vi "Control Panel.vi"(8 "error in (no error)":errorcluster, 11 "Spectrometer Digikröm.lvclass in":refnum<class "Spectrometer Digikröm.lvclass">) -> (0 "error out":errorcluster, 3 "Spectrometer Digikröm.lvclass out":refnum<class "Spectrometer Digikröm.lvclass">)   [LabVIEW 2009, in "Spectrometer Digikröm.lvclass"]
uses:
  Spectrometer Digikröm.lvclass
  <vilib>/Utility/error.llb/DialogType.ctl
  Digikrom DK24x/Digikrom DK24x.lvlib
panel:
  in  "exit":bool
  in  "Control":T1={"Goto Wavelength"=0.0, "Slit 1 width"=1.0000000000000004e-05, "Slit 2 width"=1.0000000000000004e-05, "Filter"=3, "Grating"=1} {"Grating" items=["Grating A"=1, "Grating B"=2, "Grating C"=3]; "Filter" items=["No filter", "Filter 1", "Filter 2", "Filter 3", "Filter 4", "Filter 5", ""]; "Slit 2 width" min=1.0000000000000004e-05 max=0.005000000000000002 step=1.0000000000000004e-05; "Slit 1 width" min=1.0000000000000004e-05 max=0.005000000000000002 step=1.0000000000000004e-05; "Goto Wavelength" min=0.0 max=6e-06 step=1.0000000000000008e-13 format="%.2f"}
  out "Status":T2={"Ready"=FALSE, "Wavelength"=5.000000000000003e-07, "Entrance slit"=9.999999999999999e-06, "Exit slit"=9.999999999999999e-06, " Grating (nm)"=500.0, " Filter"=0.0} {"Exit slit" format="%.2f"; "Entrance slit" format="%.2f"; "Wavelength" min=0.0 format="%.2f"}
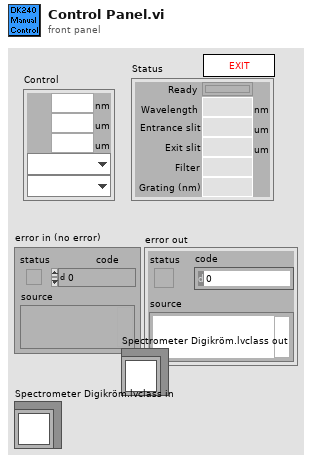
[diagram p1: front panel]
types:
  T1 = cluster{"Goto Wavelength":dbl[unit], "Slit 1 width":dbl[unit], "Slit 2 width":dbl[unit], "Filter":u32, "Grating":u16}
  T2 = cluster{"Ready":bool, "Wavelength":dbl[unit], "Entrance slit":dbl[unit], "Exit slit":dbl[unit], " Grating (nm)":dbl, " Filter":dbl}
  T3 = typedef "DialogType.ctl" = u16
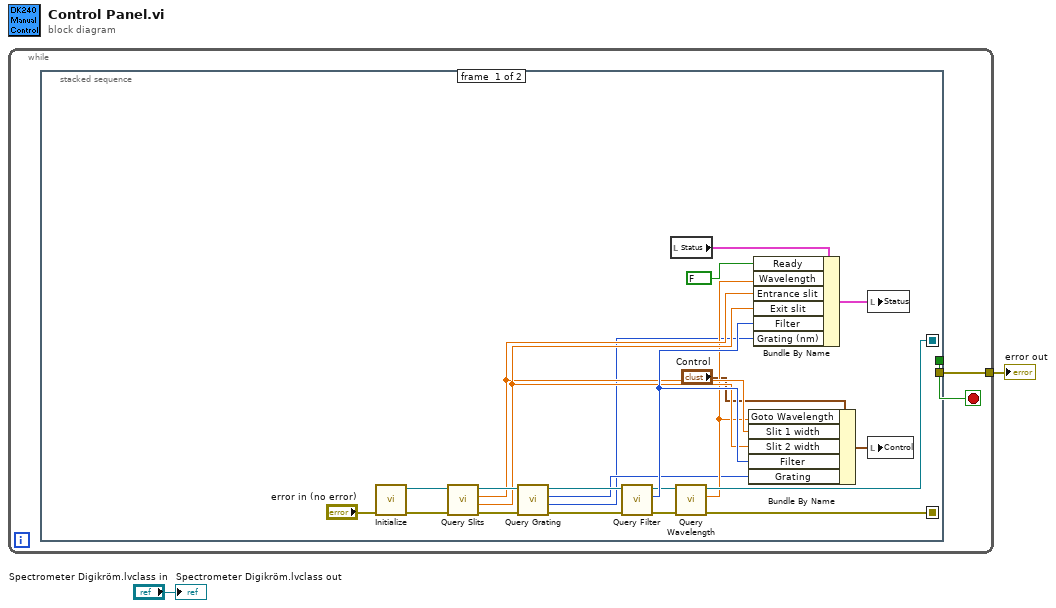
[diagram p0: block diagram]
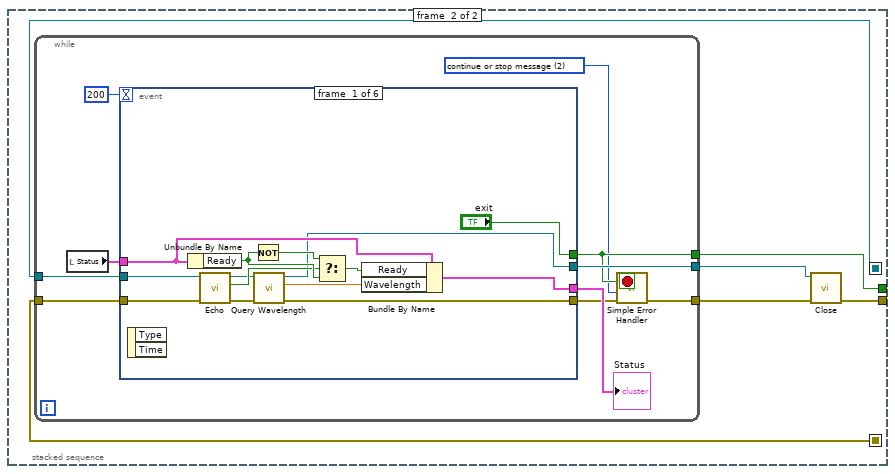
[diagram p2: hidden frame]
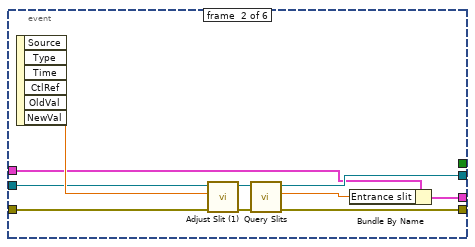
[diagram p3: hidden frame]
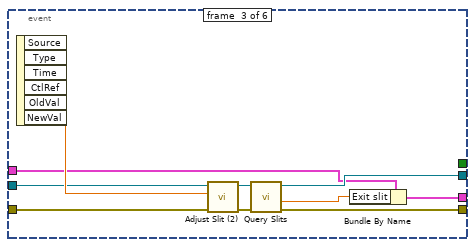
[diagram p4: hidden frame]
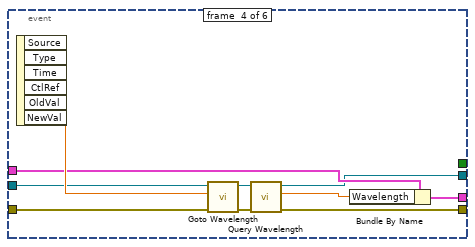
[diagram p5: hidden frame]
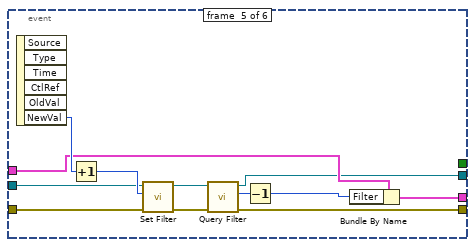
[diagram p6: hidden frame]
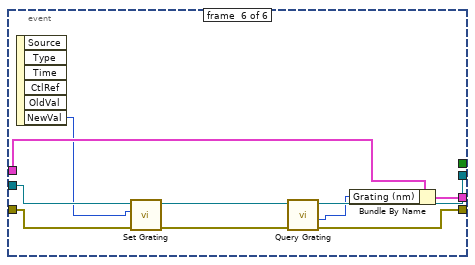
[diagram p7: hidden frame]
diagram:
  n1 = while {
    tunnel: [w3] -> w2
    stop <- w4 stop-if-true
    n2 = stacked-sequence {
      seq-local: [w19 _] -> [_ w31]
      seq-local: [w18 _] -> [_ w32]
      tunnel: [_ w30] -> w4
      tunnel: [_ w27] -> w3
      frame #0 {
        n3 = call "Initialize.vi"("error in (no error)"="error in (no error)") -> ("error out"=w23:errorcluster, "VISA resource name out"=w22:refnum<visa-resource-name>)  [unwired: 2 in, 7 out]
        n4 = call "Query Slits.vi"("error in (no error)"=w23, "VISA resource name"=w22) -> ("error out"=w20:errorcluster, "CURRENT S2 WIDTH"=w15:dbl[unit], "CURRENT S1 WIDTH"=w14:dbl[unit], "VISA resource name out"=w21:refnum<visa-resource-name>)  [unwired: 6 out]
        n5 = call "Query Grating.vi"("error in (no error)"=w20, "VISA resource name"=w21) -> ("error out"=w9:errorcluster, "BLAZE (nm)"=w7:u16, "GRATING #"=w8:u8, "VISA resource name out"=w10:refnum<visa-resource-name>)  [unwired: 6 out]
        n6 = call "Query Filter.vi"("error in (no error)"=w9, "VISA resource name"=w10) -> ("error out"=w11:errorcluster, "CURRENT FILTER"=w16:u8, "VISA resource name out"=w12:refnum<visa-resource-name>)  [unwired: 7 out]
        n7 = local read "Status"() -> (w25:T2)
        n8 = call "Query Wavelength.vi"("error in (no error)"=w11, "VISA resource name"=w12) -> ("error out"=w18:errorcluster, "CURRENT WAVELENGTH"=w13:dbl[unit], "VISA resource name out"=w19:refnum<visa-resource-name>)  [unwired: 7 out]
        n9 = Bundle By Name(cluster="Control", "Goto Wavelength"=w13, "Slit 1 width"=w14, "Slit 2 width"=w15, "Filter"=w16, "Grating"=w8) -> (w24:T1)
        n10 = Bundle By Name(cluster=w25, "Ready"=FALSE, "Wavelength"=w13, "Entrance slit"=w14, "Exit slit"=w15, "Filter"=w16, "Grating (nm)"=w7) -> (w26:T2)
        n11 = local write "Status"(w26) -> ()
        n12 = local write "Control"(w24) -> ()
      }
      frame #1 {
        n13 = while {
          tunnel: [w35] -> w30
          tunnel: w32 -> [w40]
          tunnel: [w34] -> w29
          tunnel: w31 -> [w39]
          tunnel: [w38] -> w28
          stop <- w35 stop-if-true
          w33 = T3 2 items=["no dialog", "OK message", "continue or stop message", "OK message + warnings", "continue/stop + warnings"] ("type of dialog (OK msg:1)")
          n14 = local read "Status"() -> (w36:T2)
          n15 = event shown="[5] \"Control.Grating\": Value Change" {
            selector: _ -> [_ _ _ _ _ _]
            dyn-events: _ -> [_ _ _ _ _ _]
            timeout: 200 -> [_ _ _ _ _ _]
            tunnel: ["exit" _ _ _ _ _] -> w35
            tunnel: [w56 w66 w76 w85 w97 w108] -> w42
            tunnel: w39 -> [w51 w60 w71 w82 w89 w107]
            tunnel: w40 -> [w52 w61 w72 w83 w93 w106]
            tunnel: [w46 w63 w74 w78 w87 w99] -> w37
            tunnel: [w47 w64 w75 w77 w88 w101] -> w38
            tunnel: w36 -> [w50 w59 w70 w81 w92 w105]
            event #0 {
              n16 = event-data() -> ()  [unwired: 3 out]
              n17 = Unbundle By Name(w50) -> ("Ready"=w53:bool)
              n18 = call "Echo.vi"("error in (no error)"=w52, "VISA resource name"=w51) -> ("error out"=w45:errorcluster, "Comm OK?"=w49:bool, "VISA resource name out"=w44:refnum<visa-resource-name>)  [unwired: 7 out]
              n19 = Not(x=w53) -> (.not. x?=w54:bool)
              n20 = call "Query Wavelength.vi"("error in (no error)"=w45, "VISA resource name"=w44) -> ("error out"=w46:errorcluster, "CURRENT WAVELENGTH"=w43:dbl[unit], "VISA resource name out"=w47:refnum<visa-resource-name>)  [unwired: 7 out]
              n21 = Select(t=w54, s=w49, f=w53) -> (s? t:f=w55:bool)
              n22 = Bundle By Name(cluster=w50, "Ready"=w55, "Wavelength"=w43) -> (w56:T2)
            }
            event #1 {
              n23 = event-data() -> ("NewVal"=w62:dbl[unit])  [unwired: 6 out]
              n24 = call "Adjust Slit (1).vi"("error in (no error)"=w61, "SLIT WIDTH"=w62, "VISA resource name"=w60) -> ("error out"=w58:errorcluster, "VISA resource name out"=w57:refnum<visa-resource-name>)  [unwired: 7 out]
              n25 = call "Query Slits.vi"("error in (no error)"=w58, "VISA resource name"=w57) -> ("error out"=w63:errorcluster, "CURRENT S1 WIDTH"=w65:dbl[unit], "VISA resource name out"=w64:refnum<visa-resource-name>)  [unwired: 7 out]
              n26 = Bundle By Name(cluster=w59, "Entrance slit"=w65) -> (w66:T2)
            }
            event #2 {
              n27 = event-data() -> ("NewVal"=w73:dbl[unit])  [unwired: 6 out]
              n28 = call "Adjust Slit (2).vi"("error in (no error)"=w72, "SLIT WIDTH"=w73, "VISA resource name"=w71) -> ("error out"=w69:errorcluster, "VISA resource name out"=w68:refnum<visa-resource-name>)  [unwired: 7 out]
              n29 = call "Query Slits.vi"("error in (no error)"=w69, "VISA resource name"=w68) -> ("error out"=w74:errorcluster, "CURRENT S2 WIDTH"=w67:dbl[unit], "VISA resource name out"=w75:refnum<visa-resource-name>)  [unwired: 7 out]
              n30 = Bundle By Name(cluster=w70, "Exit slit"=w67) -> (w76:T2)
            }
            event #3 {
              n31 = event-data() -> ("NewVal"=w86:dbl[unit])  [unwired: 6 out]
              n32 = call "Goto Wavelength.vi"("error in (no error)"=w83, "WAVELENGTH"=w86, "VISA resource name"=w82) -> ("error out"=w79:errorcluster, "VISA resource name out"=w80:refnum<visa-resource-name>)  [unwired: 7 out]
              n33 = call "Query Wavelength.vi"("error in (no error)"=w79, "VISA resource name"=w80) -> ("error out"=w78:errorcluster, "CURRENT WAVELENGTH"=w84:dbl[unit], "VISA resource name out"=w77:refnum<visa-resource-name>)  [unwired: 7 out]
              n34 = Bundle By Name(cluster=w81, "Wavelength"=w84) -> (w85:T2)
            }
            event #4 {
              n35 = event-data() -> ("NewVal"=w98:u32)  [unwired: 6 out]
              n36 = Increment(x=w98) -> (x+1=w96:u32)
              n37 = call "Set Filter.vi"("error in (no error)"=w93, "NEW FILTER"=w96, "VISA resource name"=w89) -> ("error out"=w90:errorcluster, "VISA resource name out"=w91:refnum<visa-resource-name>)  [unwired: 7 out]
              n38 = call "Query Filter.vi"("error in (no error)"=w90, "VISA resource name"=w91) -> ("error out"=w87:errorcluster, "CURRENT FILTER"=w94:u8, "VISA resource name out"=w88:refnum<visa-resource-name>)  [unwired: 7 out]
              n39 = Decrement(x=w94) -> (x-1=w95:u8)
              n40 = Bundle By Name(cluster=w92, "Filter"=w95) -> (w97:T2)
            }
            event #5 {
              n41 = event-data() -> ("NewVal"=w104:u16)  [unwired: 6 out]
              n42 = call "Set Grating.vi"("error in (no error)"=w106, "NEW GRT?"=w104, "VISA resource name"=w107) -> ("error out"=w103:errorcluster, "VISA resource name out"=w102:refnum<visa-resource-name>)  [unwired: 7 out]
              n43 = call "Query Grating.vi"("error in (no error)"=w103, "VISA resource name"=w102) -> ("error out"=w99:errorcluster, "BLAZE (nm)"=w100:u16, "VISA resource name out"=w101:refnum<visa-resource-name>)  [unwired: 7 out]
              n44 = Bundle By Name(cluster=w105, "Grating (nm)"=w100) -> (w108:T2)
            }
          }
          "Status" <- w42
          n45 = call <vilib>:"Simple Error Handler.vi"("type of dialog (OK msg:1)"=w33, "error in (no error)"=w37) -> ("error out"=w34:errorcluster)  [unwired: 7 out]
        }
        n46 = call "Close.vi"("error in (no error)"=w29, "VISA resource name"=w28) -> ("error out"=w27:errorcluster)  [unwired: 9 out]
      }
    }
  }
  "error out" <- w2
  "Spectrometer Digikröm.lvclass out" <- "Spectrometer Digikröm.lvclass in"
